vi "Handle Player.vi"(8 "Move Info":T4, 10 "Relative Seconds":dbl, 11 "Temp DVR":refnum<data-value>) -> (0 "Penalty":i32, 3 "Temp DVR":refnum<data-value>)   [LabVIEW 2015, in "SquareBattle Arena.lvlib" / "SquareBattle Arena.lvclass"]
uses:
  SquareBattle Arena.lvclass
  Runner Cluster.ctl
  Square/Square.lvclass
  Action Enum.ctl
  Direction Enum.ctl
panel:
  # "NOTICE - YOU MUST NOT REMOVE THIS NOTICE. PER THE FOLLOWING LICENSE, YOU MAY REPRODUCE THIS SOFTWARE PROVIDED YOU FOLLOW THE TERMS\nOF THE LICENSE.\n\n---BEGIN BSD LICENSE (http://opensource.org/licenses/BSD-2-Clause)---\nCopyright (c) 2015, Endigit, Inc. <robert@endigit.com>\nAll rights reserved.\n\nRedistribution and use in source and binary forms, with or without modification, are permitted provided that the following conditions are met:\n\n1. Redistributions of source code must retain the above copyright notice, this list of conditions and the following disclaimer.\n\n2. Redistributions in binary form must reproduce the above copyright notice, this list of conditions and the following disclaimer in the documentation and/or other \nmaterials provided with the distribution.\n\nTHIS SOFTWARE IS PROVIDED BY THE COPYRIGHT HOLDERS AND CONTRIBUTORS \"AS IS\" AND ANY EXPRESS OR IMPLIED WARRANTIES, INCLUDING, BUT NOT \nLIMITED TO, THE IMPLIED WARRANTIES OF MERCHANTABILITY AND FITNESS FOR A PARTICULAR PURPOSE ARE DISCLAIMED. IN NO EVENT SHALL THE COPYRIGHT \nHOLDER OR CONTRIBUTORS BE LIABLE FOR ANY DIRECT, INDIRECT, INCIDENTAL, SPECIAL, EXEMPLARY, OR CONSEQUENTIAL DAMAGES (INCLUDING, BUT NOT \nLIMITED TO, PROCUREMENT OF SUBSTITUTE GOODS OR SERVICES; LOSS OF USE, DATA, OR PROFITS; OR BUSINESS INTERRUPTION) HOWEVER CAUSED AND ON \nANY THEORY OF LIABILITY, WHETHER IN CONTRACT, STRICT LIABILITY, OR TORT (INCLUDING NEGLIGENCE OR OTHERWISE) ARISING IN ANY WAY OUT OF THE USE \nOF THIS SOFTWARE, EVEN IF ADVISED OF THE POSSIBILITY OF SUCH DAMAGE.\n---END BSD LICENSE---"
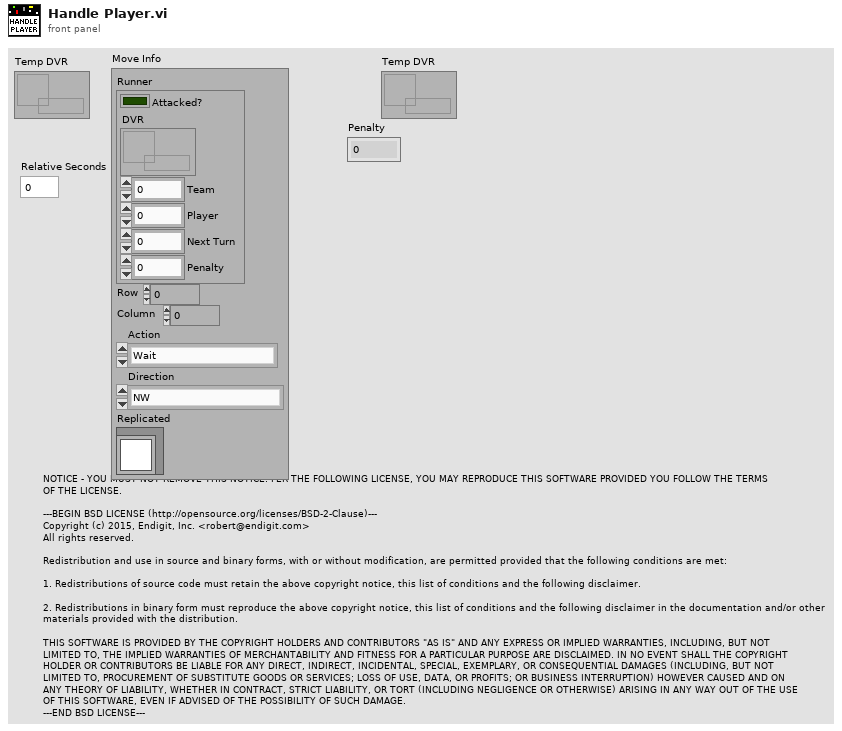
[diagram p1: front panel]
types:
  T1 = typedef "SquareBattle Arena.lvlib/SquareBattle Arena.lvclass/Runner Cluster.ctl" = cluster{"Attacked?":bool, "DVR":refnum<data-value>, "Team":i32, "Player":i32, "Next Turn":i32, "Penalty":i32}
  T2 = typedef "SquareBattle Arena.lvlib/SquareBattle Arena.lvclass/Action Enum.ctl" = enum16{"Wait", "Move", "Attack", "Replicate"}
  T3 = typedef "SquareBattle Arena.lvlib/SquareBattle Arena.lvclass/Direction Enum.ctl" = enum16{"NW", "N", "NE", "E", "SE", "S", "SW", "W"}
  T4 = cluster{"Runner":T1, "Row":i32, "Column":i32, "Action":T2, "Direction":T3, "Replicated":refnum<class "Square.lvclass">}
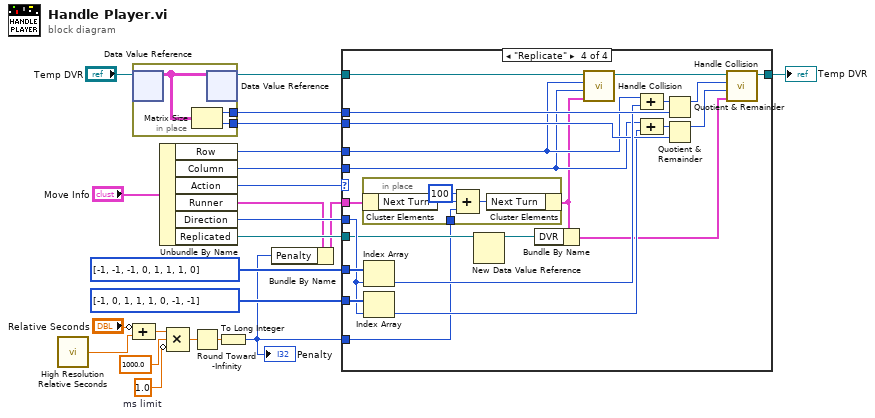
[diagram p0: block diagram]
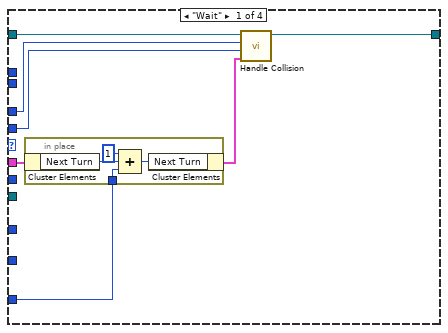
[diagram p2: hidden frame]
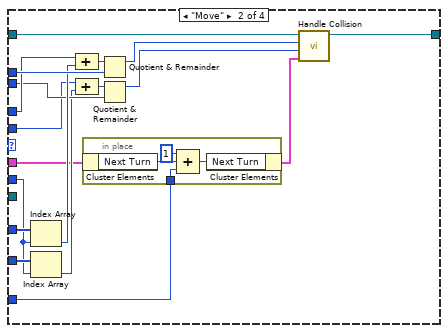
[diagram p3: hidden frame]
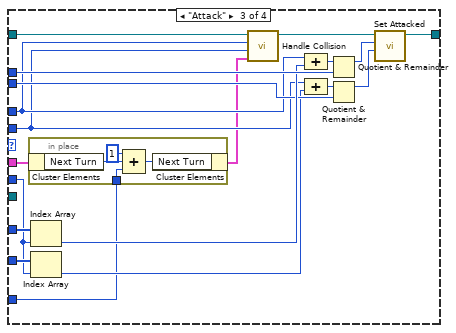
[diagram p4: hidden frame]
diagram:
  w4 = 1.0  # ms limit
  n1 = call <vilib>:"High Resolution Relative Seconds.vi"() -> ("relative seconds"=w10:dbl)
  n2 = in-place {
    in-place-border: [w25] -> w19
    in-place-border: [w24] -> w18
    n3 = in-place-dvr #1("Temp DVR") -> (w26:T1[][])  [unwired: 1 out]
    n4 = Matrix Size(0:w26) -> (1:w25:i32, 2:w24:i32)
    n5 = in-place-dvr #1(w26) -> (w20:refnum<data-value>)  [unwired: 1 out]
  }
  n6 = Compound Arithmetic op=ADD(invert "Relative Seconds", w10) -> (w8:dbl)
  n7 = Unbundle By Name("Move Info") -> ("Row"=w17:i32, "Column"=w16:i32, "Action"=w23:T2, "Runner"=w3:T1, "Direction"=w15:T3, "Replicated"=w14:refnum<class "Square.lvclass">)
  n8 = Compound Arithmetic op=MULTIPLY(w8, 1000.0 ("value"), invert w4) -> (w7:dbl)
  n9 = Round Toward -Infinity(1:w7) -> (0:w6:dbl)
  n10 = To Long Integer(number=w6) -> (32bit integer=w1:i32)
  "Penalty" <- w1
  n11 = Bundle By Name(cluster=w3, "Penalty"=w1) -> (w2:T1)
  n12 = case shown="\"Replicate\"" w23 {
    tunnel: w20 -> [w33 w55 w78 w104]
    tunnel: w19 -> [_ w50 w73 w99]
    tunnel: w18 -> [_ w45 w70 w96]
    tunnel: w17 -> [w32 w48 w68 w94]
    tunnel: w16 -> [w31 w43 w67 w93]
    tunnel: w2 -> [w29 w40 w62 w85]
    tunnel: w15 -> [_ w52 w75 w101]
    tunnel: i32[] [-1, -1, -1, 0, 1, 1, 1, 0] -> [_ w54 w77 w103]
    tunnel: i32[] [-1, 0, 1, 1, 1, 0, -1, -1] -> [_ w53 w76 w102]
    tunnel: w14 -> [_ _ _ w86]
    tunnel: [w30 w41 w63 w87] -> w13
    tunnel: w1 -> [w27 w38 w61 w83]
    frame "Wait" {
      n13 = in-place {
        in-place-border: w27 -> [w35]
        n14 = in-place-cluster #2(w29) -> ("Next Turn"=w37:i32)
        n15 = Compound Arithmetic op=ADD(1 ("value"), w37, w35) -> (w36:i32)
        n16 = in-place-cluster #2("Next Turn"=w36) -> (w28:T1)
      }
      n17 = call "Handle Collision.vi"("Cluster"=w28, "Column"=w31, "Row"=w32, "Temp DVR"=w33) -> ("Temp DVR"=w30:refnum<data-value>)  [unwired: 7 in]
    }
    frame "Move" {
      n18 = Index Array(array=w54, index=w52) -> (element=w47:i32)
      n19 = Index Array(array=w53, index=w52) -> (element=w42:i32)
      n20 = Compound Arithmetic op=ADD(w48, w47) -> (w51:i32)
      n21 = Compound Arithmetic op=ADD(w43, w42) -> (w46:i32)
      n22 = in-place {
        in-place-border: w38 -> [w57]
        n23 = in-place-cluster #3(w40) -> ("Next Turn"=w59:i32)
        n24 = Compound Arithmetic op=ADD(1 ("value"), w59, w57) -> (w58:i32)
        n25 = in-place-cluster #3("Next Turn"=w58) -> (w39:T1)
      }
      n26 = Quotient & Remainder(x=w51, y=w50) -> (x-y*floor(x/y)=w49:i32)  [unwired: 1 out]
      n27 = Quotient & Remainder(x=w46, y=w45) -> (x-y*floor(x/y)=w44:i32)  [unwired: 1 out]
      n28 = call "Handle Collision.vi"("Cluster"=w39, "Column"=w44, "Row"=w49, "Temp DVR"=w55) -> ("Temp DVR"=w41:refnum<data-value>)  [unwired: 7 in]
    }
    frame "Attack" {
      n29 = in-place {
        in-place-border: w61 -> [w80]
        n30 = in-place-cluster #4(w62) -> ("Next Turn"=w82:i32)
        n31 = Compound Arithmetic op=ADD(1 ("value"), w82, w80) -> (w81:i32)
        n32 = in-place-cluster #4("Next Turn"=w81) -> (w60:T1)
      }
      n33 = Index Array(array=w77, index=w75) -> (element=w72:i32)
      n34 = Index Array(array=w76, index=w75) -> (element=w69:i32)
      n35 = call "Handle Collision.vi"("Cluster"=w60, "Column"=w67, "Row"=w68, "Temp DVR"=w78) -> ("Temp DVR"=w66:refnum<data-value>)  [unwired: 7 in]
      n36 = Compound Arithmetic op=ADD(w68, w72) -> (w74:i32)
      n37 = Compound Arithmetic op=ADD(w67, w69) -> (w71:i32)
      n38 = Quotient & Remainder(x=w74, y=w73) -> (x-y*floor(x/y)=w65:i32)  [unwired: 1 out]
      n39 = Quotient & Remainder(x=w71, y=w70) -> (x-y*floor(x/y)=w64:i32)  [unwired: 1 out]
      n40 = call "Set Attacked.vi"("Column"=w64, "Row"=w65, "Temp DVR"=w66) -> ("Temp DVR"=w63:refnum<data-value>)  [unwired: 8 in]
    }
    frame "Replicate" {
      n41 = in-place {
        in-place-border: w83 -> [w106]
        n42 = in-place-cluster #5(w85) -> ("Next Turn"=w108:i32)
        n43 = Compound Arithmetic op=ADD(100 ("value"), w108, w106) -> (w107:i32)
        n44 = in-place-cluster #5("Next Turn"=w107) -> (w84:T1)
      }
      n45 = Index Array(array=w103, index=w101) -> (element=w98:i32)
      n46 = Index Array(array=w102, index=w101) -> (element=w95:i32)
      n47 = New Data Value Reference(data value=w86) -> (data value reference=w89:refnum<data-value>)  [unwired: 1 in, 1 out]
      n48 = Bundle By Name(cluster=w84, "DVR"=w89) -> (w88:T1)
      n49 = call "Handle Collision.vi"("Cluster"=w84, "Column"=w93, "Row"=w94, "Temp DVR"=w104) -> ("Temp DVR"=w92:refnum<data-value>)  [unwired: 7 in]
      n50 = Compound Arithmetic op=ADD(w94, w98) -> (w100:i32)
      n51 = Compound Arithmetic op=ADD(w93, w95) -> (w97:i32)
      n52 = Quotient & Remainder(x=w100, y=w99) -> (x-y*floor(x/y)=w91:i32)  [unwired: 1 out]
      n53 = Quotient & Remainder(x=w97, y=w96) -> (x-y*floor(x/y)=w90:i32)  [unwired: 1 out]
      n54 = call "Handle Collision.vi"("Cluster"=w88, "Column"=w90, "Row"=w91, "Temp DVR"=w92) -> ("Temp DVR"=w87:refnum<data-value>)  [unwired: 7 in]
    }
  }
  "Temp DVR" <- w13
